vi "ObjectTable.vi"(8 "ObjectStoreSelector":T1(ring), 11 "Name":string) -> (0 "ObjectTable":cluster{"Name":string, "ObjectRef":refnum<vi>}[](array[cluster]), 1 "UniqueName":string, 2 "ObjectRefArray":refnum<vi>[](array[refnum]), 3 "ObjectRef":refnum<vi>, 4 "Names":string[](array[string]))   [LabVIEW 2014]
uses:
  <vilib>/picture/3D Picture Control/Object/Create Object (name).vi
  <vilib>/picture/3D Picture Control/NI_3D Picture Control.lvlib
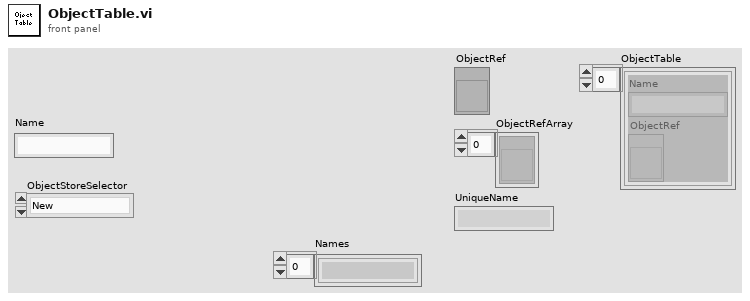
[diagram p1: front panel]
types:
  T1 = enum16{"New", "Find", "FindPattern", "GetTable", "Clear"}
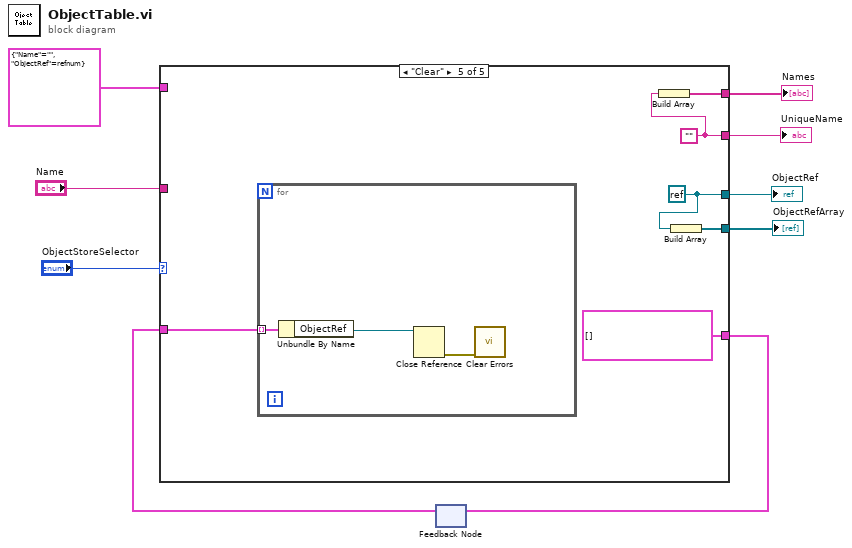
[diagram p0: block diagram]
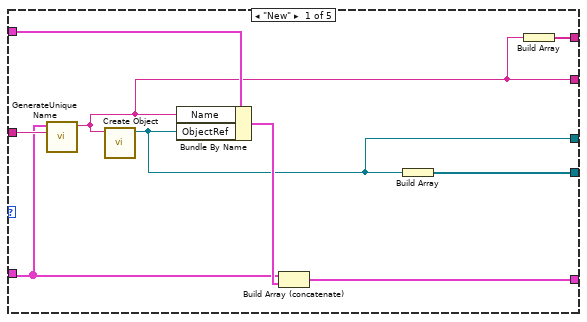
[diagram p2: hidden frame]
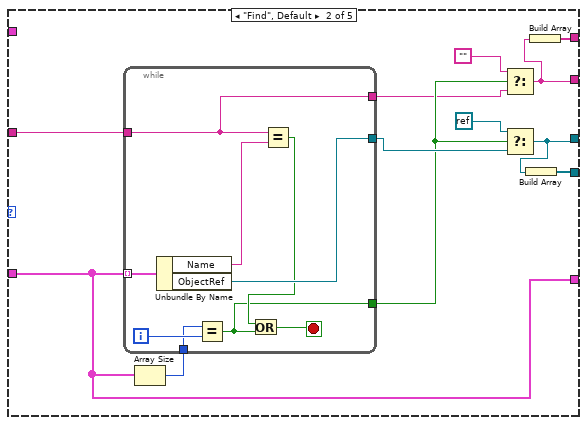
[diagram p3: hidden frame]
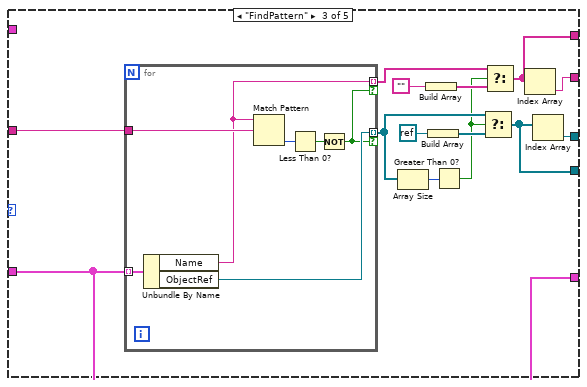
[diagram p4: hidden frame]
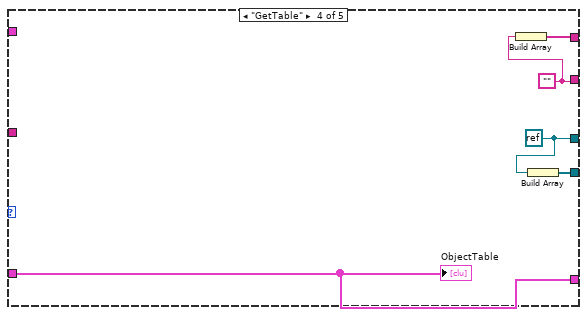
[diagram p5: hidden frame]
diagram:
  n1 = feedback #1() -> (w8:cluster{"Name":string, "ObjectRef":refnum<vi>}[])  [unwired: 1 in]
  n2 = case shown="\"Clear\"" "ObjectStoreSelector" {
    tunnel: w8 -> [w12 w29 w46 w63 w71]
    tunnel: "Name" -> [w13 w30 w53 _ _]
    tunnel: cluster{"Name":string, "ObjectRef":refnum<vi>} {"Name"="", "ObjectRef"=refnum} -> [w18 _ _ _ _]
    tunnel: [w16 w29 w46 w63 cluster{"Name":string, "ObjectRef":refnum<vi>}[] []] -> w5
    tunnel: [w15 w25 w49 w64 w69] -> w4
    tunnel: [w14 w24 w50 w65 w70] -> w3
    tunnel: [w11 w20 w41 w62 w68] -> w2
    tunnel: [w10 w19 w40 w61 w67] -> w1
    frame "New" {
      n3 = call "GenerateUniqueName.vi"("Name"=w13, "ObjectTable"=w12) -> ("UniqueName"=w11:string)  [unwired: 9 in]
      n4 = call-poly <vilib>:"Create Object.vi"("Name"=w11) -> ("Scene:New Object"=w15:refnum<vi>)  [unwired: 9 in, 1 out]
      n5 = Bundle By Name(cluster=w18, "Name"=w11, "ObjectRef"=w15) -> (w17:cluster{"Name":string, "ObjectRef":refnum<vi>})
      n6 = Build Array (concatenate)(w12, w17) -> (w16:cluster{"Name":string, "ObjectRef":refnum<vi>}[])
      n7 = Build Array(w15) -> (w14:refnum<vi>[])
      n8 = Build Array(w11) -> (w10:string[])
    }
    frame "Find", Default {
      n9 = Array Size(array=w29) -> (size(s)=w28:i32)
      n10 = while {
        tunnel: w29 -> [w39] mode=indexing
        tunnel: w30 -> [w31]
        tunnel: [w37] -> w27
        tunnel: w28 -> [w35]
        tunnel: [w32] -> w23
        tunnel: [w31] -> w21
        i -> [w36]
        stop <- w33 stop-if-true
        n11 = Unbundle By Name(w39) -> ("Name"=w38:string, "ObjectRef"=w37:refnum<vi>)
        n12 = Equal?(x=w35, y=w36) -> (x = y?=w32:bool)
        n13 = Equal?(x=w31, y=w38) -> (x = y?=w34:bool)
        n14 = Or(x=w34, y=w32) -> (x .or. y?=w33:bool)
      }
      n15 = Select(t="", s=w23, f=w21) -> (s? t:f=w20:string)
      n16 = Select(t=refnum<k0> refnum, s=w23, f=w27) -> (s? t:f=w25:refnum<vi>)
      n17 = Build Array(w25) -> (w24:refnum<vi>[])
      n18 = Build Array(w20) -> (w19:string[])
    }
    frame "FindPattern" {
      n19 = for {
        tunnel: w46 -> [w60] mode=indexing
        tunnel: w53 -> [w58]
        tunnel: [w59] -> w51 mode=indexing if=w54
        tunnel: [w55] -> w42 mode=indexing if=w54
        n20 = Unbundle By Name(w60) -> ("Name"=w55:string, "ObjectRef"=w59:refnum<vi>)
        n21 = Match Pattern(string=w55, regular expression=w58) -> (offset past match=w57:i32)  [unwired: 1 in, 3 out]
        n22 = Less Than 0?(x=w57) -> (x < 0?=w56:bool)
        n23 = Not(x=w56) -> (.not. x?=w54:bool)
      }
      n24 = Array Size(array=w51) -> (size(s)=w52:i32)
      n25 = Build Array("") -> (w44:string[])
      n26 = Build Array(refnum<k0> refnum) -> (w47:refnum<k0>[])
      n27 = Greater Than 0?(x=w52) -> (x > 0?=w43:bool)
      n28 = Select(t=w51, s=w43, f=w47) -> (s? t:f=w50:refnum<vi>[])
      n29 = Select(t=w42, s=w43, f=w44) -> (s? t:f=w40:string[])
      n30 = Index Array(array=w40) -> (element=w41:string)  [unwired: 1 in]
      n31 = Index Array(array=w50) -> (element=w49:refnum<vi>)  [unwired: 1 in]
    }
    frame "GetTable" {
      w62 = ""
      w64 = refnum<k0> refnum
      n32 = Build Array(w62) -> (w61:string[])
      n33 = Build Array(w64) -> (w65:refnum<k0>[])
      "ObjectTable" <- w63
    }
    frame "Clear" {
      w68 = ""
      w69 = refnum<k0> refnum
      n34 = for {
        tunnel: w71 -> [w74] mode=indexing
        n35 = Unbundle By Name(w74) -> ("ObjectRef"=w73:refnum<vi>)
        n36 = Close Reference(reference=w73) -> (error out=w72:errorcluster)  [unwired: 1 in]
        n37 = call <vilib>:"Clear Errors.vi"("error in (no error)"=w72) -> ()  [unwired: 5 in, 2 out]
      }
      n38 = Build Array(w68) -> (w67:string[])
      n39 = Build Array(w69) -> (w70:refnum<k0>[])
    }
  }
  "ObjectRef" <- w4
  "ObjectRefArray" <- w3
  "UniqueName" <- w2
  "Names" <- w1
  n40 = feedback-in #1(w5) -> ()
